vi "Clear NULL.vi"(11 "Type in":refnum<class "Type.lvclass">) -> (3 "Type out":refnum<class "Type.lvclass">)   [LabVIEW 2020, in "Conditum.lvlib" / "Columns.lvlib" / "Type.lvclass"]
uses:
  Type.lvclass
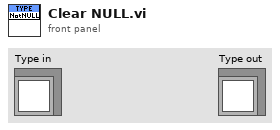
[diagram p1: front panel]
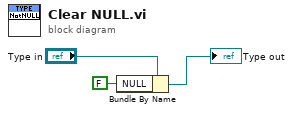
[diagram p0: block diagram]
diagram:
  n1 = Bundle By Name(cluster="Type in", "NULL"=FALSE) -> (→"Type out":refnum<class "Type.lvclass">)
